vi "Read Data and Search for Property Value.vi"() -> ()   [LabVIEW 2012]
uses:
  <vilib>/Utility/file.llb/Read From Spreadsheet File (string).vi
panel:
  in  "属性名":string="UUT序列号"
  out "属性值":string
  out "数组形式的电子表格文件":string[][](array[string])
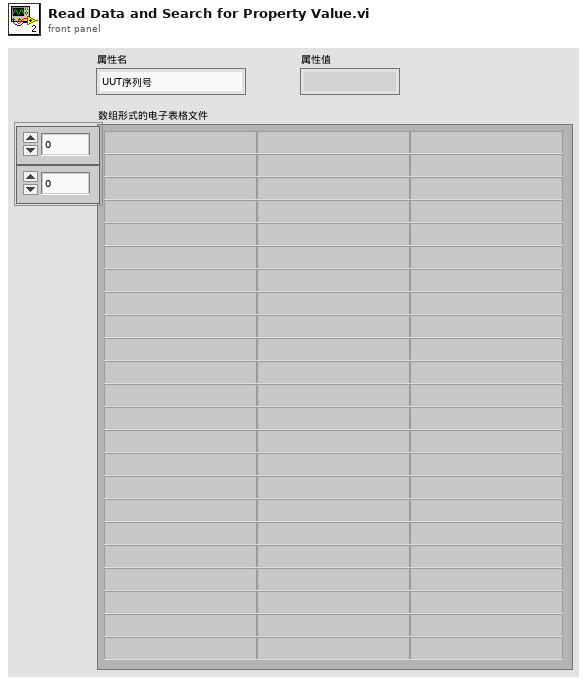
[diagram p1: front panel]
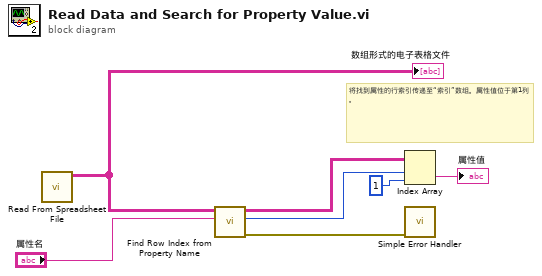
[diagram p0: block diagram]
diagram:
  # "将找到属性的行索引传递至“索引”数组。属性值位于第1列。"
  n1 = call-poly <vilib>:"Read From Spreadsheet File.vi"() -> ("all rows"=w7:string[][])  [unwired: 7 in, 4 out]
  "数组形式的电子表格文件" <- w7
  n2 = call "Find Row Index from Property Name.vi"("属性名"="属性名", "电子表格字符串数组"=w7) -> ("错误输出"=w1:cluster{"状态":bool, "代码":i32, "源":string}, "行索引"=w6:i32, "电子表格字符串数组输出"=w5:string[][])  [unwired: 7 in]
  n3 = Index Array ("索引数组")(array=w5, index (row)=w6, index (col)=1 ("长度")) -> (element=→"属性值":string)
  n4 = call <vilib>:"Simple Error Handler.vi"("error in (no error)"=w1) -> ()  [unwired: 4 in, 5 out]
